vi "Connect.vi"(8 "error in":errorcluster, 11 "6700 in":refnum<class "6700.lvclass">) -> (0 "error out":errorcluster, 3 "6700 out":refnum<class "6700.lvclass">)   [LabVIEW 2018, in "6700.lvlib" / "6700.lvclass"]
uses:
  6700.lvclass
  <instrlib>/Agilent N6700 Series/Agilent N6700 Series.lvlib
  builds/Power_Supply.lvlibp/Power Supply.lvclass
  C:/Users/Ron.Dexter.LUMINARTECH/Desktop/builds/Power_Supply.lvlibp/Power Supply.lvclass
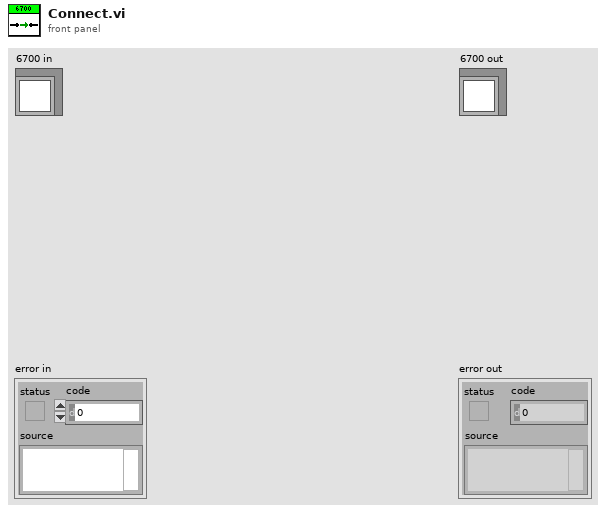
[diagram p1: front panel]
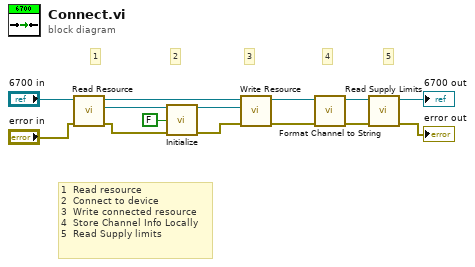
[diagram p0: block diagram]
diagram:
  # "5"
  # "4"
  # "1  Read resource\n2  Connect to device\n3  Write connected resource\n4  Store Channel Info Locally\n5  Read Supply limits"
  # "3"
  # "2"
  # "1"
  n1 = call "Read Resource.vi"("error in"="error in", "Power Supply in"="6700 in") -> ("error out"=w11:errorcluster, "Resource"=w12:refnum<visa-resource-name>, "Power Supply out"=w8:refnum<class "6700.lvclass">)  [unwired: 7 in]
  n2 = call <instrlib>:"Initialize.vi"("VISA resource name"=w12, "Reset? (T: Yes)"=FALSE, "error in (no error)"=w11) -> ("VISA resource name out"=w9:refnum<visa-resource-name>, "error out"=w7:errorcluster)  [unwired: 11 in]
  n3 = call "Write Resource.vi"("error in"=w7, "Resource"=w9, "Power Supply in"=w8) -> ("error out"=w3:errorcluster, "Power Supply out"=w4:refnum<class "6700.lvclass">)  [unwired: 7 in]
  n4 = call "Format Channel to String.vi"("error in"=w3, "6700 in"=w4) -> ("error out"=w2:errorcluster, "6700 out"=w1:refnum<class "6700.lvclass">)  [unwired: 8 in]
  n5 = call "Read Supply Limits.vi"("error in"=w2, "6700 in"=w1) -> ("error out"=→"error out":errorcluster, "6700 out"=→"6700 out":refnum<class "6700.lvclass">)  [unwired: 8 in]
